vi "DSF.Shared.Configuration.Transfer.From Object.vi"(8 "error in (no error)":errorcluster, 10 "object":refnum<class>, 11 "Transfer Configuration in":refnum<class "DSF.Shared.Configuration.Transfer.lvclass">) -> (0 "error out":errorcluster, 2 "default class used?":bool, 3 "Transfer Configuration out":refnum<class "DSF.Shared.Configuration.Transfer.lvclass">)   [LabVIEW 2017, in "DSF.Shared.lvlib" / "DSF.Shared.Configuration.Transfer.lvclass"]
uses:
  DSF.Shared.Configuration.Transfer.lvclass
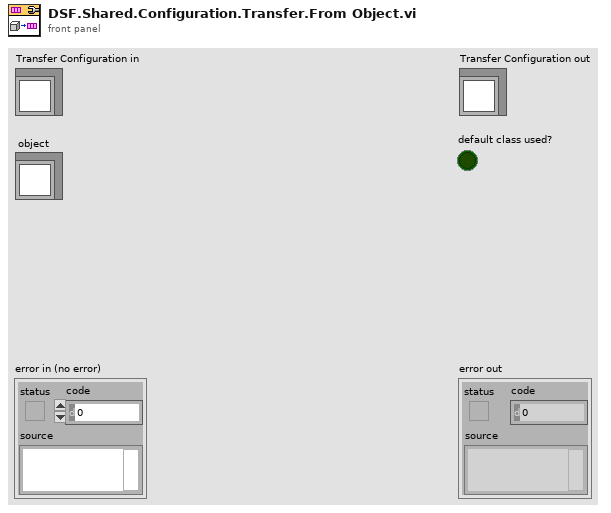
[diagram p1: front panel]
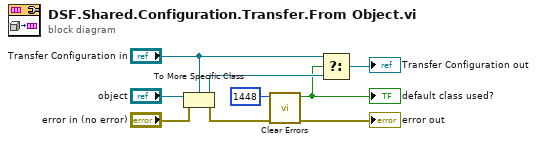
[diagram p0: block diagram]
diagram:
  n1 = To More Specific Class(target class="Transfer Configuration in", reference="object", error in="error in (no error)") -> (specific class reference=w7:refnum<class "DSF.Shared.Configuration.Transfer.lvclass">, error out=w8:errorcluster)
  n2 = call <vilib>:"Clear Errors.vi"("error in (no error)"=w8, "specific error code to clear (0: all)"=1448) -> ("error out"=→"error out":errorcluster, "specific error cleared?"=w1:bool)  [unwired: 4 in]
  "default class used?" <- w1
  n3 = Select(t="Transfer Configuration in", s=w1, f=w7) -> (s? t:f=→"Transfer Configuration out":refnum<class "DSF.Shared.Configuration.Transfer.lvclass">)
